vi "R45.vi"() -> ()   [LabVIEW 2016]
uses:
  <vilib>/Instr/_visa.llb/VISA Open Access Mode.ctl
  save load/SaveLoad.lvlib
  save load/saveloadprev.ctl
panel:
  in  "Tab Control":T1(tab)
  out "X Mag steerer":bool=TRUE
  out "ExB 2":bool
  in  "GFM set (Amps)":dbl(slide) min=0.0 max=150.0 scale=0.0..100.0
  in  "ExB #2 Electric":dbl(slide) min=0.0 max=200.0 scale=0.0..40.0
  in  "Reset ExB 2":bool
  in  "ExB #1 Electric":dbl(slide) min=0.0 max=200.0 scale=0.0..46.0
  out "R45 Steerer Y Read":dbl format="%#.2g"
  out "R45 Steerer X Read":dbl format="%#.2g"
  in  "R45 Y steerer":dbl(slide) min=-10.0 max=10.0 scale=-10.0..8.0
  in  "R45 Quad A":dbl(slide) min=0.0 max=200.0 scale=10.0..120.0
  in  "R45 X steerer":dbl(slide) min=-10.0 max=10.0 scale=-10.0..10.0
  out "R45 Steerer":bool
  out "R45 quad Range":bool
  in  "R45 Quad B":dbl(slide) min=0.0 max=200.0 scale=50.0..80.0
  in  "stop":bool
  out "ExB 1":bool
  out "ExB Voltage Read-":dbl format="%#.2g"
  in  "ExB #1 Magnet":dbl(slide) scale=0.0..10.0
  out "ExB Voltage Read +":dbl format="%#.2g"
  out "read current quad B":string
  out "read voltage quad B":string
  out "read current quad A":string
  out "read voltage Quad A":string
  in  "R45 X steerer end":dbl(slide) min=-10.0 max=10.0 scale=-10.0..10.0
  in  "ExB #2 Magnet":dbl(slide) scale=0.0..10.0
  out "GFM read":string
  out "r45 end x steerer read":dbl
  in  "Preview-Save-Load":T2
  out "ExB#1 +READ I":dbl
  out "ExB - I":dbl
  in  "R45 temp file":path=path "D:/Main Tune Parameters/Temp Configs/R45.txt"
  in  "Quad A VISA GPIB Resource":refnum<visa-resource-name>="GPIB1::6::INSTR"
  in  "Quad B VISA GPIB Resource":refnum<visa-resource-name>="GPIB1::3::INSTR"
  out "SV error":errorcluster
  out "Quad B error":errorcluster
  out "Quad A error":errorcluster
  out "GFM SV error":errorcluster
  out "SaveLoad error":errorcluster
  # "R45"
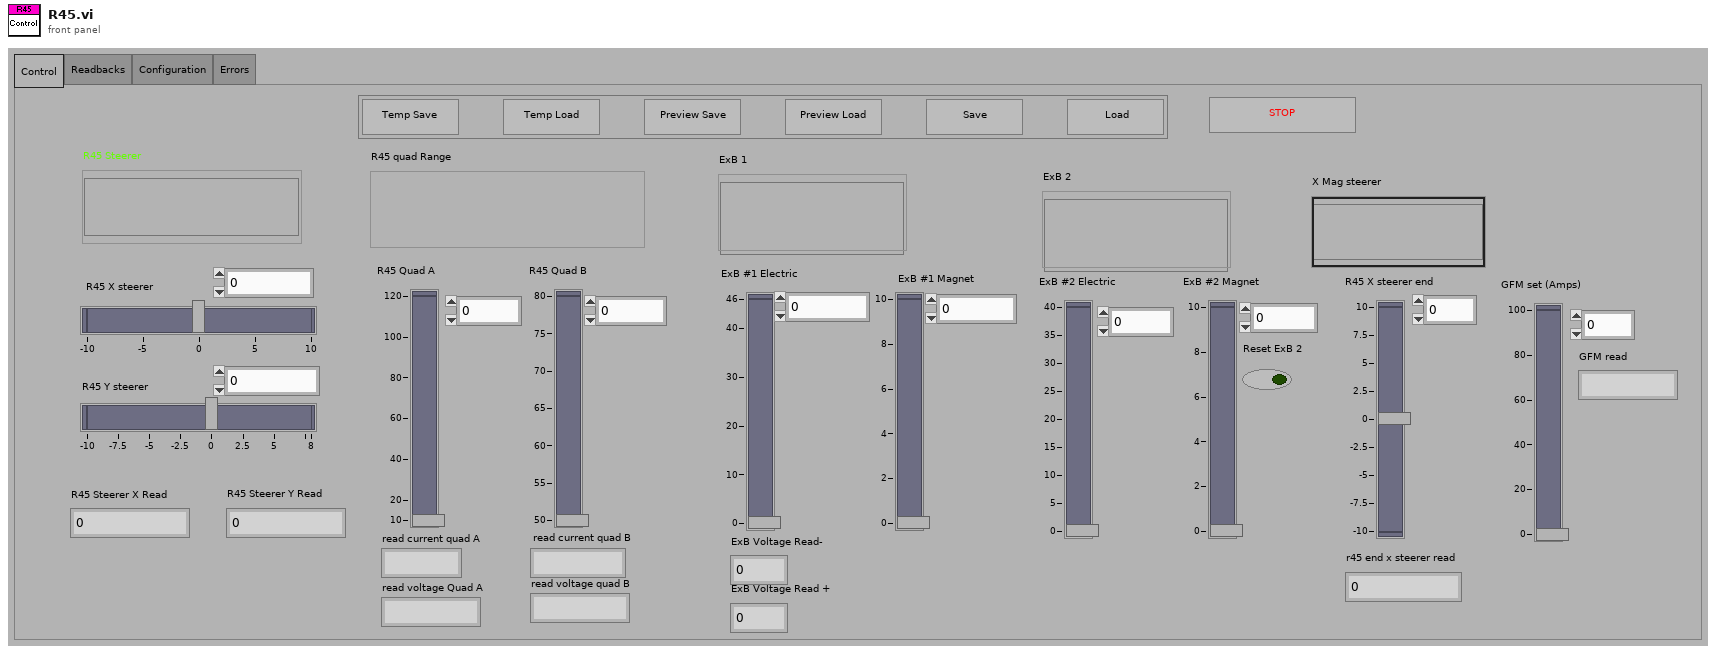
[diagram p1: front panel]
types:
  T1 = enum32{"Control", "Readbacks", "Configuration", "Errors"}
  T2 = typedef "saveloadprev.ctl" = cluster{"Temp Save":bool, "Temp Load":bool, "Save":bool, "Load":bool, "Preview Save":bool, "Preview Load":bool}
  T3 = typedef "VISA Open Access Mode.ctl" = u32
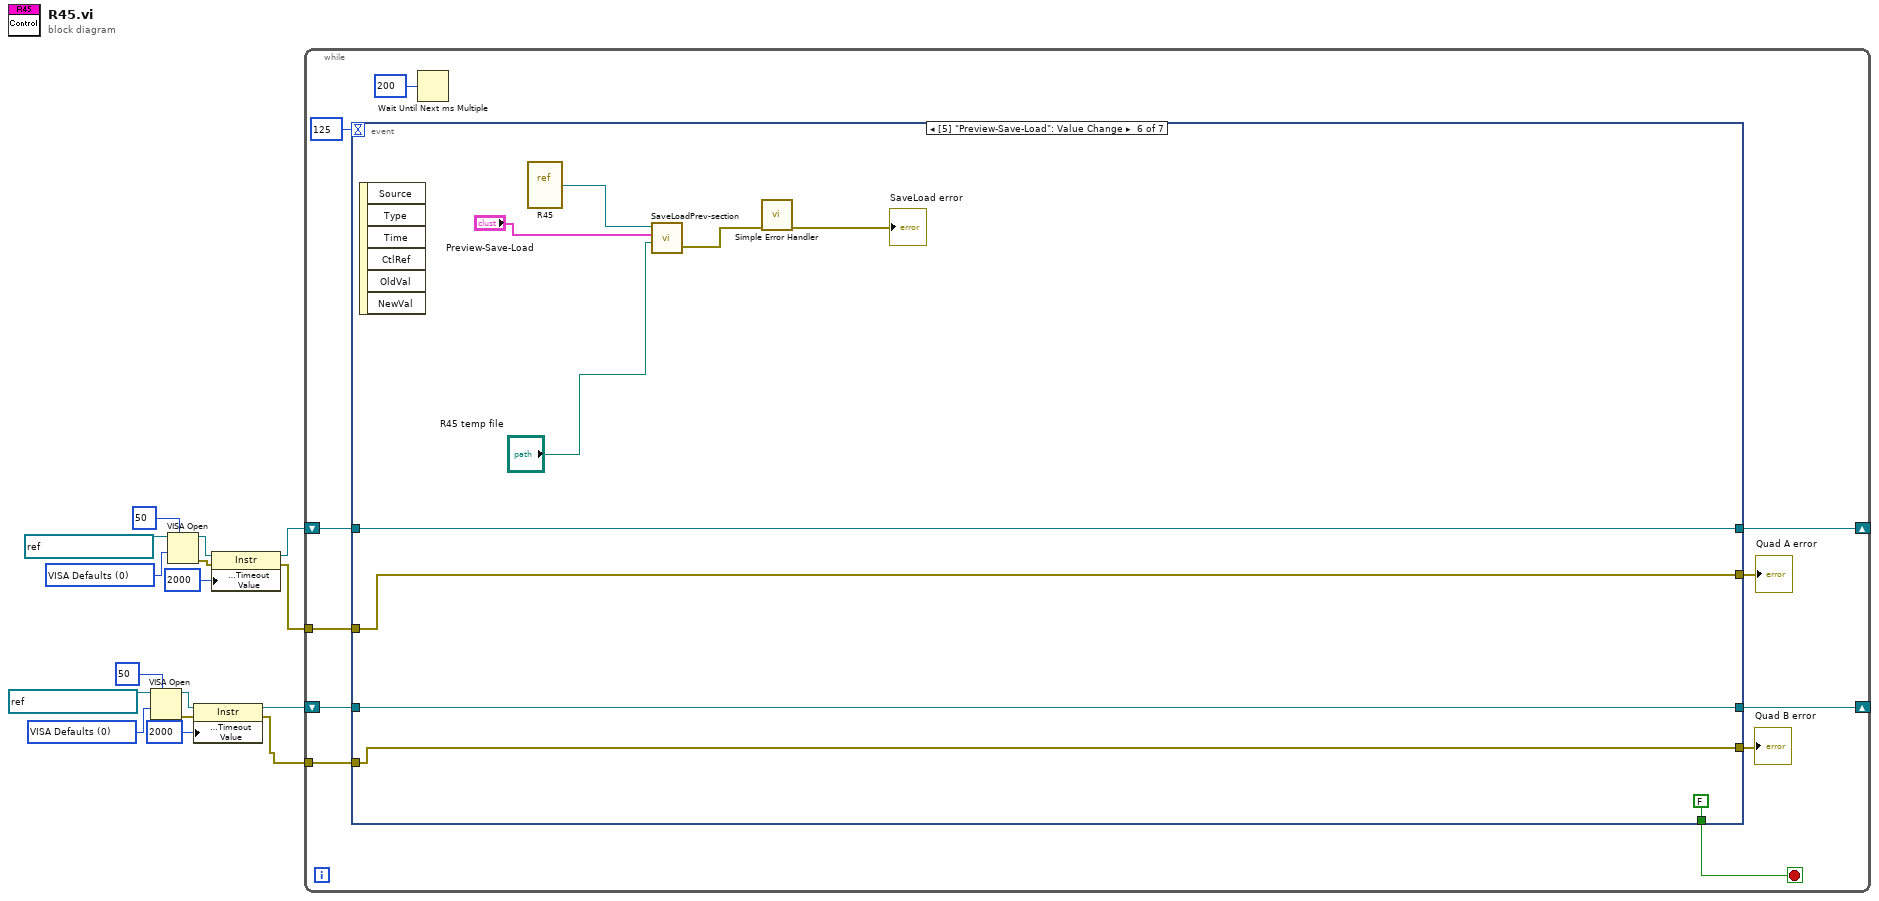
[diagram p0: block diagram]
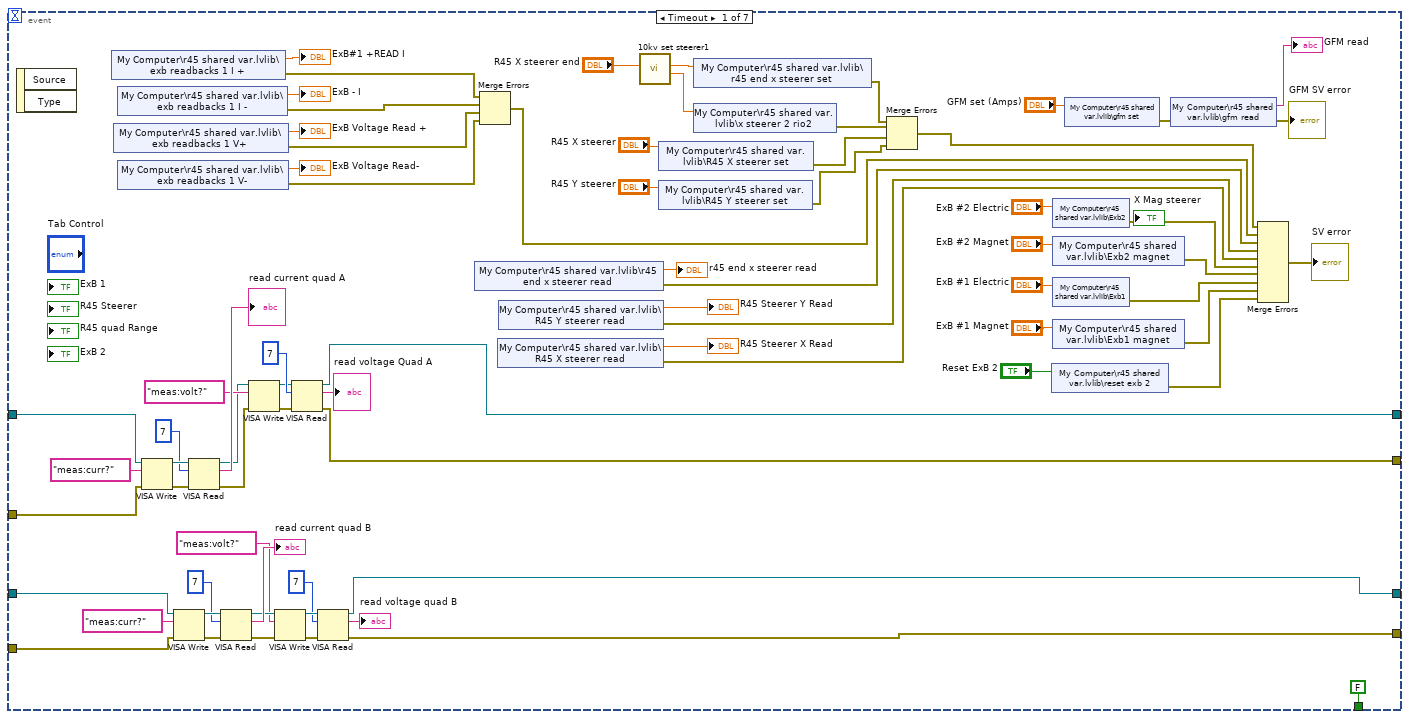
[diagram p2: hidden frame]
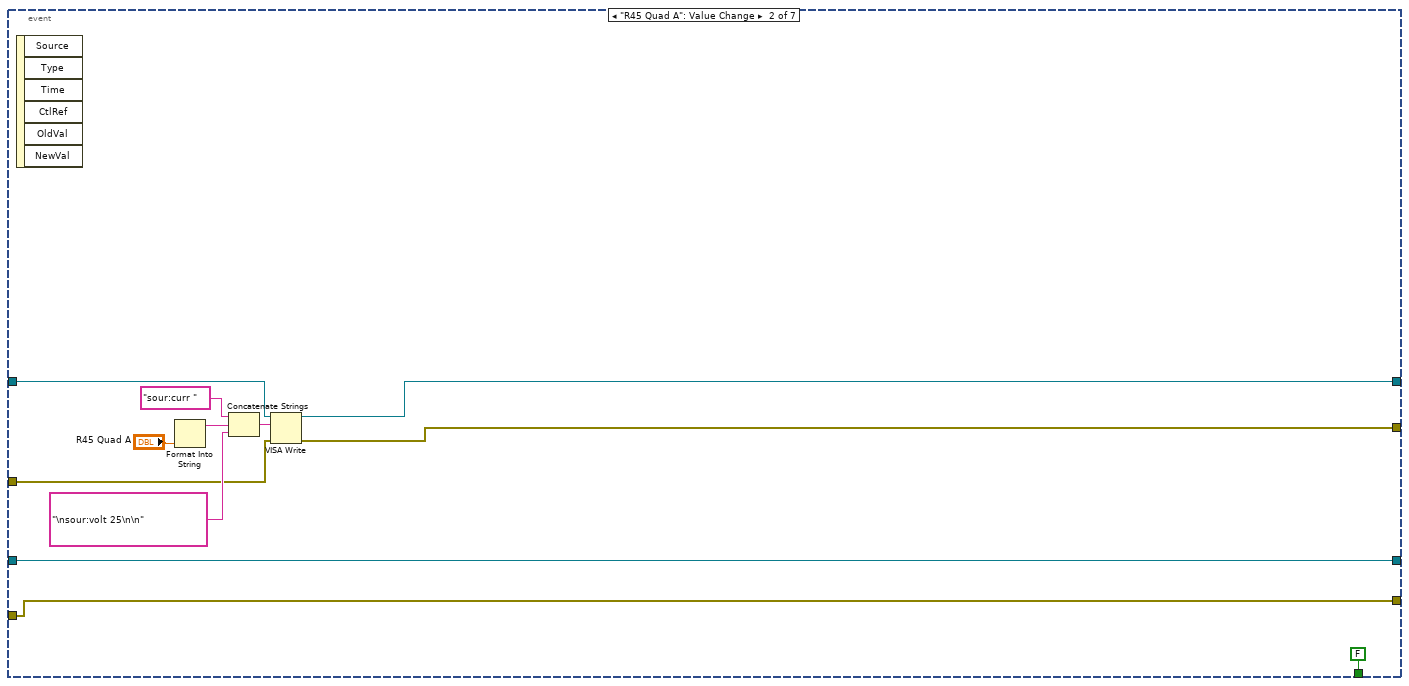
[diagram p3: hidden frame]
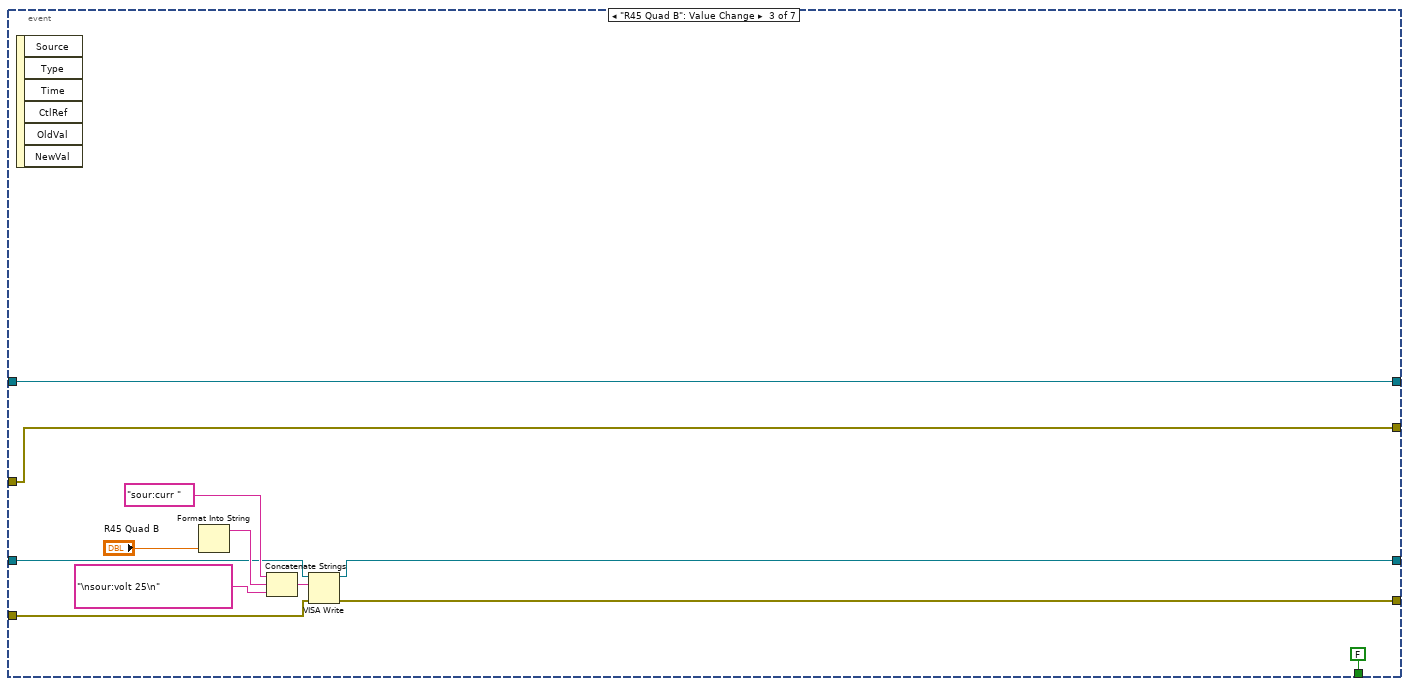
[diagram p4: hidden frame]
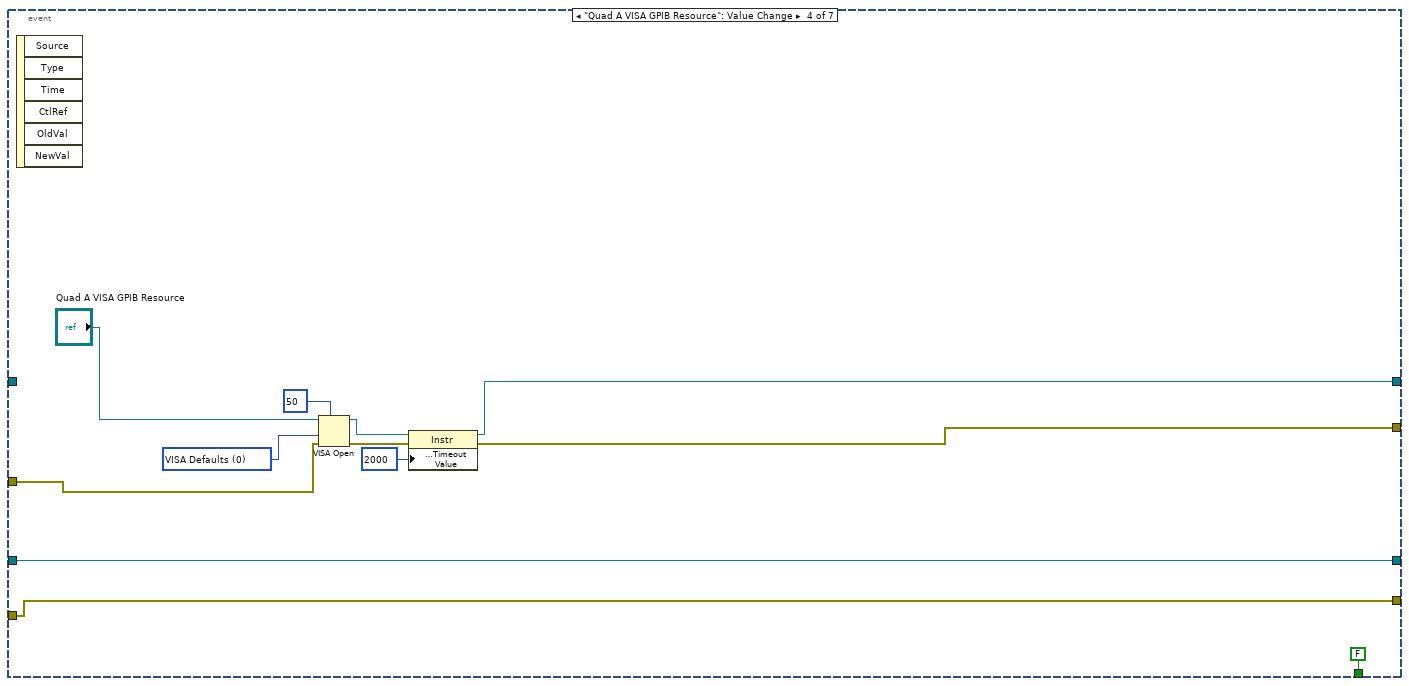
[diagram p5: hidden frame]
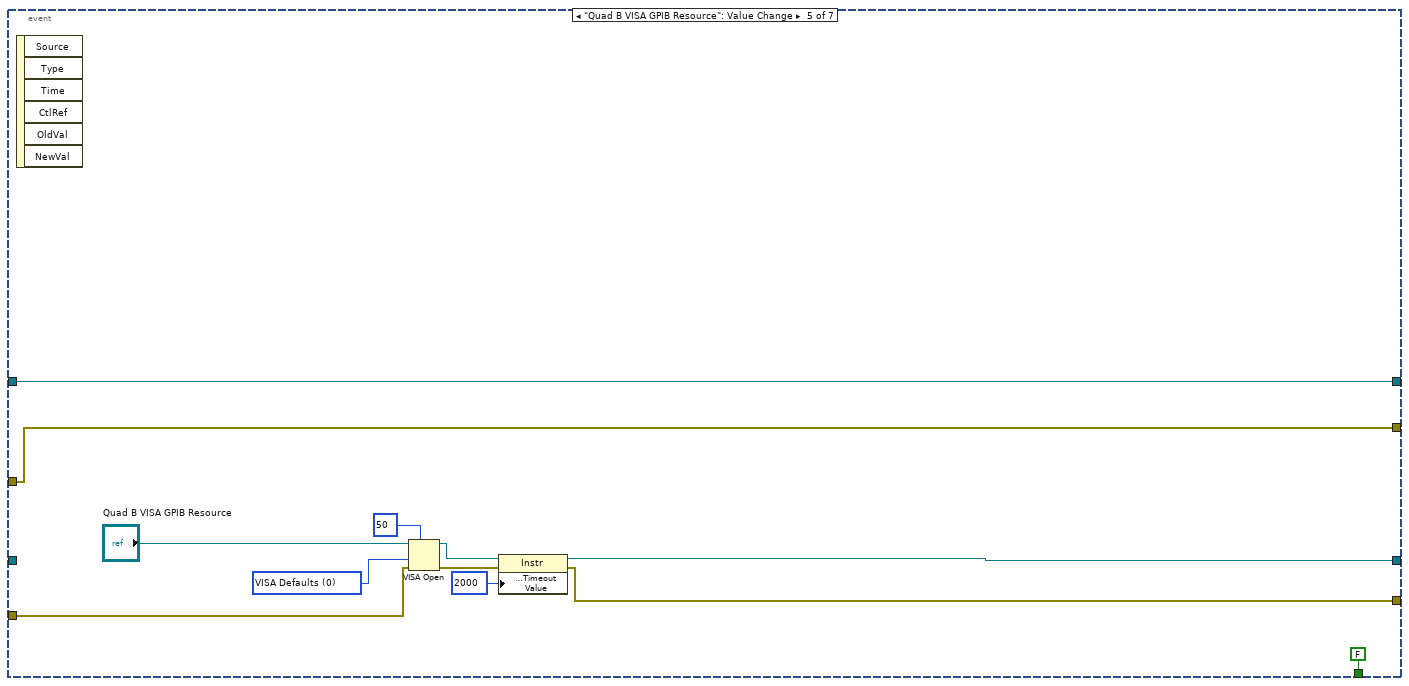
[diagram p6: hidden frame]
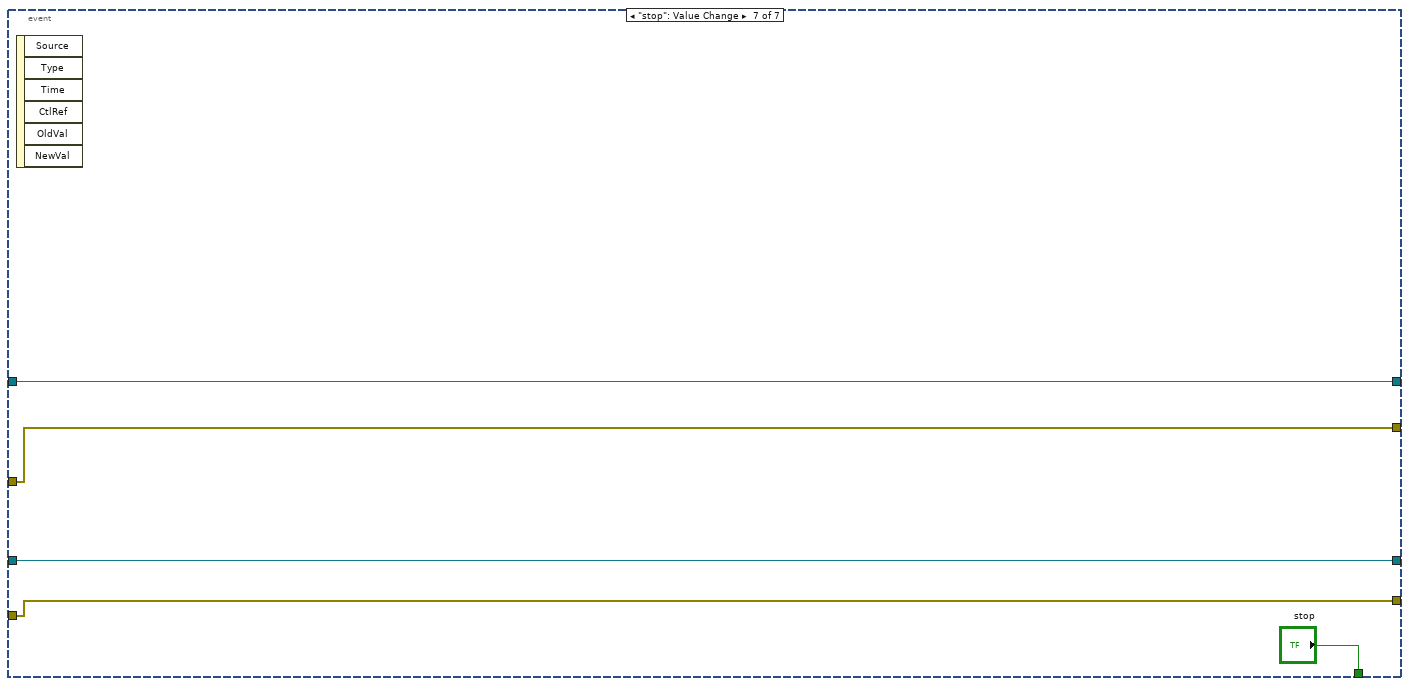
[diagram p7: hidden frame]
diagram:
  w15 = T3 0 items=["VISA Defaults"=0, "Exclusive Lock"=1, "Load Configured Settings"=4] ("Access Mode")
  w6 = T3 0 items=["VISA Defaults"=0, "Exclusive Lock"=1, "Load Configured Settings"=4] ("Access Mode")
  n1 = VISA Open(timeout (0)=u32 50 ("VISA Open timeout (0)"), access mode=w6, VISA resource name=refnum<visa-resource-name> "GPIB1::6::INSTR" ("VISA GPIB Resource")) -> (VISA resource name=w10:refnum<visa-resource-name>, error out=w11:errorcluster)  [unwired: 2 in]
  n2 = VISA Open(timeout (0)=u32 50 ("VISA Open timeout (0)"), access mode=w15, VISA resource name=refnum<visa-resource-name> "GPIB1::3::INSTR" ("VISA GPIB Resource")) -> (VISA resource name=w1:refnum<visa-resource-name>, error out=w12:errorcluster)  [unwired: 2 in]
  n3 = property class="Instr"(reference=w10, error in=w11, "General Settings:Timeout Value"=u32 2000) -> (reference out=w2:refnum<visa-resource-name>, error out=w3:errorcluster)
  n4 = property class="Instr"(reference=w1, error in=w12, "General Settings:Timeout Value"=u32 2000) -> (reference out=w5:refnum<visa-resource-name>, error out=w4:errorcluster)
  n5 = while {
    tunnel: w4 -> [w25]
    tunnel: w3 -> [w23]
    shift-right: [w20] -> _
    shift-left: w2 -> [w22]
    shift-right: [w19] -> _
    shift-left: w5 -> [w26]
    stop <- w27 stop-if-true
    n6 = event shown="[5] \"Preview-Save-Load\": Value Change" {
      selector: _ -> [_ _ _ _ _ _ _]
      dyn-events: _ -> [_ _ _ _ _ _ _]
      timeout: 125 -> [_ _ _ _ _ _ _]
      tunnel: [FALSE ("stop") FALSE ("stop") FALSE ("stop") FALSE ("stop") FALSE ("stop") FALSE ("stop") "stop"] -> w27
      tunnel: w26 -> [w71 w106 w113 _ w137 w157 w159]
      tunnel: w25 -> [w72 w105 w114 w130 w138 w156 w160]
      tunnel: [w70 w103 w114 w127 w138 w156 w160] -> w24
      tunnel: w23 -> [w86 w101 w118 w125 w142 w154 w161]
      tunnel: w22 -> [w87 w102 w117 w126 _ w155 w162]
      tunnel: [w85 w101 w116 w125 w139 w154 w161] -> w21
      tunnel: [w28 w102 w115 w126 w140 w155 w162] -> w20
      tunnel: [w69 w104 w113 w128 w137 w157 w159] -> w19
      event Timeout {
        n7 = event-data() -> ()  [unwired: 1 in, 2 out]
        n8 = shared-variable "My Computer\\r45 shared var.lvlib\\exb readbacks 1 I +"() -> (→"ExB#1 +READ I":dbl, error out=w38:errorcluster)  [unwired: 1 in]
        n9 = shared-variable "My Computer\\r45 shared var.lvlib\\exb readbacks 1 V+"() -> (→"ExB Voltage Read +":dbl, error out=w36:errorcluster)  [unwired: 1 in]
        n10 = shared-variable "My Computer\\r45 shared var.lvlib\\exb readbacks 1 I -"() -> (→"ExB - I":dbl, error out=w37:errorcluster)  [unwired: 1 in]
        n11 = shared-variable "My Computer\\r45 shared var.lvlib\\exb readbacks 1 V-"() -> (→"ExB Voltage Read-":dbl, error out=w35:errorcluster)  [unwired: 1 in]
        n12 = VISA Write(VISA resource name=w71, write buffer="meas:curr?" ("string"), error in (no error)=w72) -> (VISA resource name out=w83:refnum<visa-resource-name>, error out=w73:errorcluster)  [unwired: 1 out]
        n13 = VISA Write(VISA resource name=w87, write buffer="meas:curr?" ("string"), error in (no error)=w86) -> (VISA resource name out=w98:refnum<visa-resource-name>, error out=w99:errorcluster)  [unwired: 1 out]
        n14 = VISA Read(VISA resource name=w83, byte count=u32 7, error in (no error)=w73) -> (VISA resource name out=w78:refnum<visa-resource-name>, read buffer=→"read current quad A":string, error out=w74:errorcluster)  [unwired: 1 out]
        n15 = VISA Read(VISA resource name=w98, byte count=u32 7, error in (no error)=w99) -> (VISA resource name out=w91:refnum<visa-resource-name>, read buffer=→"read current quad B":string, error out=w90:errorcluster)  [unwired: 1 out]
        n16 = VISA Write(VISA resource name=w78, write buffer="meas:volt?", error in (no error)=w74) -> (VISA resource name out=w76:refnum<visa-resource-name>, error out=w80:errorcluster)  [unwired: 1 out]
        n17 = VISA Write(VISA resource name=w91, write buffer="meas:volt?", error in (no error)=w90) -> (VISA resource name out=w93:refnum<visa-resource-name>, error out=w88:errorcluster)  [unwired: 1 out]
        n18 = VISA Read(VISA resource name=w76, byte count=u32 7, error in (no error)=w80) -> (VISA resource name out=w69:refnum<visa-resource-name>, read buffer=→"read voltage Quad A":string, error out=w70:errorcluster)  [unwired: 1 out]
        n19 = VISA Read(VISA resource name=w93, byte count=u32 7, error in (no error)=w88) -> (VISA resource name out=w28:refnum<visa-resource-name>, read buffer=→"read voltage quad B":string, error out=w85:errorcluster)  [unwired: 1 out]
        n20 = shared-variable "My Computer\\r45 shared var.lvlib\\r45 end x steerer read"() -> (→"r45 end x steerer read":dbl, error out=w39:errorcluster)  [unwired: 1 in]
        n21 = Merge Errors(w38, w37, w36, w35) -> (w34:errorcluster)
        n22 = shared-variable "My Computer\\r45 shared var.lvlib\\R45 X steerer read"() -> (→"R45 Steerer X Read":dbl, error out=w41:errorcluster)  [unwired: 1 in]
        n23 = shared-variable "My Computer\\r45 shared var.lvlib\\R45 Y steerer read"() -> (→"R45 Steerer Y Read":dbl, error out=w40:errorcluster)  [unwired: 1 in]
        n24 = call "10kv set steerer1.vi"("Steerer Control IN"="R45 X steerer end") -> ("- Steerer"=w49:dbl, "+ Steerer"=w48:dbl)  [unwired: 8 in, 1 out]
        n25 = shared-variable "My Computer\\r45 shared var.lvlib\\R45 X steerer set"("R45 X steerer") -> (error out=w30:errorcluster)  [unwired: 1 in]
        n26 = shared-variable "My Computer\\r45 shared var.lvlib\\R45 Y steerer set"("R45 Y steerer") -> (error out=w29:errorcluster)  [unwired: 1 in]
        n27 = shared-variable "My Computer\\r45 shared var.lvlib\\r45 end x steerer set"(w48) -> (error out=w32:errorcluster)  [unwired: 1 in]
        n28 = shared-variable "My Computer\\r45 shared var.lvlib\\x steerer 2 rio2"(w49) -> (error out=w31:errorcluster)  [unwired: 1 in]
        n29 = Merge Errors(w32, w31, w30, w29) -> (w33:errorcluster)
        n30 = shared-variable "My Computer\\r45 shared var.lvlib\\reset exb 2"("Reset ExB 2") -> (error out=w46:errorcluster)  [unwired: 1 in]
        n31 = shared-variable "My Computer\\r45 shared var.lvlib\\Exb2"("ExB #2 Electric") -> (error out=w42:errorcluster)  [unwired: 1 in]
        n32 = shared-variable "My Computer\\r45 shared var.lvlib\\Exb2 magnet"("ExB #2 Magnet") -> (error out=w43:errorcluster)  [unwired: 1 in]
        n33 = shared-variable "My Computer\\r45 shared var.lvlib\\Exb1"("ExB #1 Electric") -> (error out=w44:errorcluster)  [unwired: 1 in]
        n34 = shared-variable "My Computer\\r45 shared var.lvlib\\Exb1 magnet"("ExB #1 Magnet") -> (error out=w45:errorcluster)  [unwired: 1 in]
        n35 = shared-variable "My Computer\\r45 shared var.lvlib\\gfm set"("GFM set (Amps)") -> (error out=w67:errorcluster)  [unwired: 1 in]
        n36 = shared-variable "My Computer\\r45 shared var.lvlib\\gfm read"(error in=w67) -> (→"GFM read":string, error out=→"GFM SV error":errorcluster)
        n37 = Merge Errors(w33, w34, w39, w40, w41, w42, w43, w44, w45, w46) -> (→"SV error":errorcluster)
      }
      event "R45 Quad A": Value Change {
        n38 = event-data() -> ()  [unwired: 1 in, 6 out]
        n39 = Format Into String("R45 Quad A") -> (resulting string=w107:string)  [unwired: 3 in, 1 out]
        n40 = Concatenate Strings("sour:curr " ("string"), w107, "\nsour:volt 25\n\n" ("write buffer")) -> (w108:string)
        n41 = VISA Write(VISA resource name=w106, write buffer=w108, error in (no error)=w105) -> (VISA resource name out=w104:refnum<visa-resource-name>, error out=w103:errorcluster)  [unwired: 1 out]
      }
      event "R45 Quad B": Value Change {
        n42 = event-data() -> ()  [unwired: 1 in, 6 out]
        n43 = Format Into String("R45 Quad B") -> (resulting string=w119:string)  [unwired: 3 in, 1 out]
        n44 = Concatenate Strings("sour:curr " ("string"), w119, "\nsour:volt 25\n" ("write buffer")) -> (w121:string)
        n45 = VISA Write(VISA resource name=w117, write buffer=w121, error in (no error)=w118) -> (VISA resource name out=w115:refnum<visa-resource-name>, error out=w116:errorcluster)  [unwired: 1 out]
      }
      event "Quad A VISA GPIB Resource": Value Change {
        w134 = T3 0 items=["VISA Defaults"=0, "Exclusive Lock"=1, "Load Configured Settings"=4] ("Access Mode")
        n46 = event-data() -> ()  [unwired: 1 in, 6 out]
        n47 = VISA Open(timeout (0)=u32 50 ("VISA Open timeout (0)"), access mode=w134, error in (no error)=w130, VISA resource name="Quad A VISA GPIB Resource") -> (VISA resource name=w132:refnum<visa-resource-name>, error out=w131:errorcluster)  [unwired: 1 in]
        n48 = property class="Instr"(reference=w132, error in=w131, "General Settings:Timeout Value"=u32 2000) -> (reference out=w128:refnum<visa-resource-name>, error out=w127:errorcluster)
      }
      event "Quad B VISA GPIB Resource": Value Change {
        w146 = T3 0 items=["VISA Defaults"=0, "Exclusive Lock"=1, "Load Configured Settings"=4] ("Access Mode")
        n49 = event-data() -> ()  [unwired: 1 in, 6 out]
        n50 = VISA Open(timeout (0)=u32 50 ("VISA Open timeout (0)"), access mode=w146, error in (no error)=w142, VISA resource name="Quad B VISA GPIB Resource") -> (VISA resource name=w144:refnum<visa-resource-name>, error out=w143:errorcluster)  [unwired: 1 in]
        n51 = property class="Instr"(reference=w144, error in=w143, "General Settings:Timeout Value"=u32 2000) -> (reference out=w140:refnum<visa-resource-name>, error out=w139:errorcluster)
      }
      event Value Change {
        n52 = event-data() -> ()  [unwired: 1 in, 6 out]
        n53 = vi-ref "R45.vi"() -> (w152:refnum<vi>)
        n54 = call "SaveLoadPrev-section.vi"("file path (use dialog)"="R45 temp file", "Cluster 2"="Preview-Save-Load", "VI Refnum"=w152) -> ("error out"=w150:errorcluster)  [unwired: 2 in]
        n55 = call <vilib>:"Simple Error Handler.vi"("error in (no error)"=w150) -> ("error out"=→"SaveLoad error":errorcluster)  [unwired: 4 in, 4 out]
      }
      event "stop": Value Change {
        n56 = event-data() -> ()  [unwired: 1 in, 6 out]
      }
    }
    "Quad A error" <- w24
    "Quad B error" <- w21
    n57 = Wait Until Next ms Multiple(millisecond multiple=u32 200) -> ()  [unwired: 1 out]
  }
